vi "autoMaintainCurrentInstructions.vi"(6 "error in (no error)":errorcluster, 7 "MotionProfile acceleration":dbl[](array[numeric]), 8 "MotionProfile speed":dbl[](array[numeric]), 9 "running commands":string[][](array[string])) -> (0 "error out":errorcluster, 3 "running commands out":string[][](array[string]))   [LabVIEW 2013]
panel:
  out "BasicDriveOffset":dbl=1.07
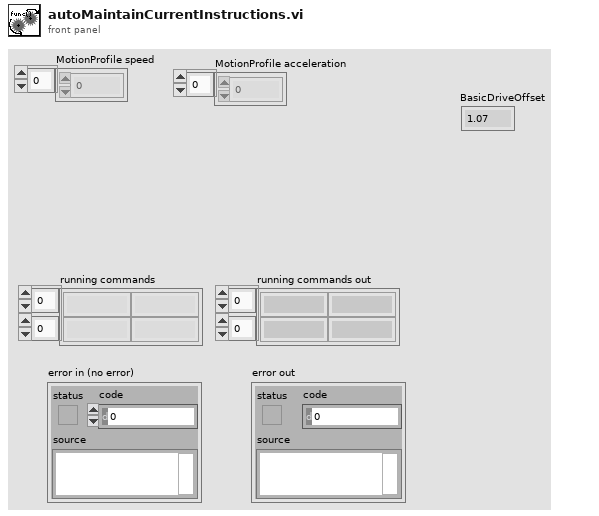
[diagram p1: front panel]
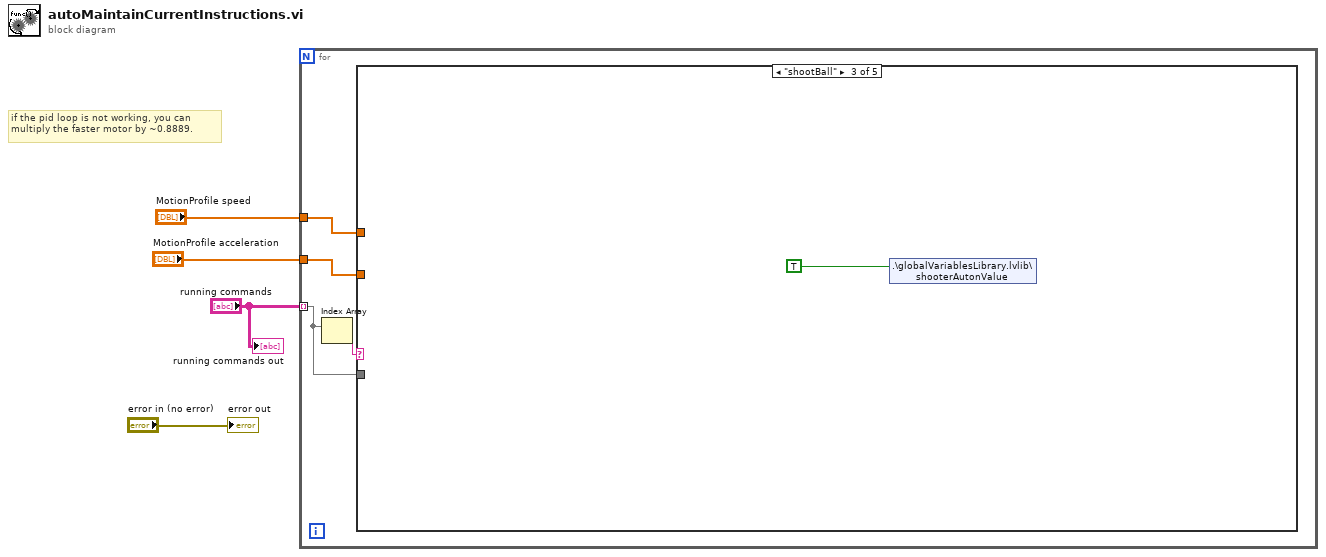
[diagram p0: block diagram]
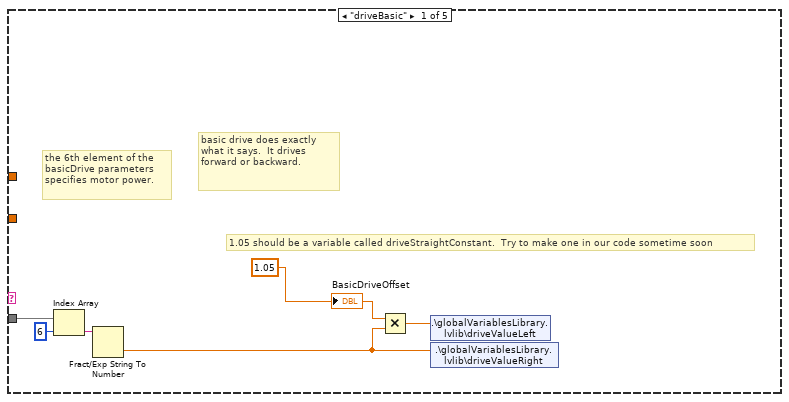
[diagram p2: hidden frame]
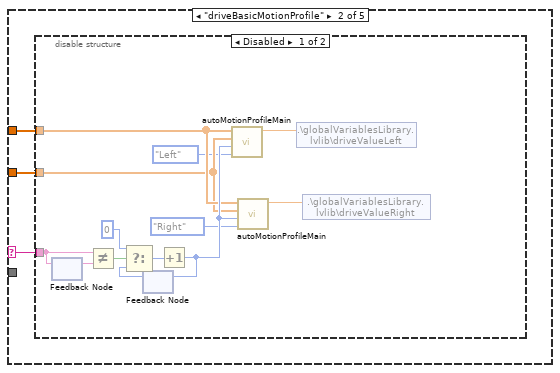
[diagram p3: hidden frame]
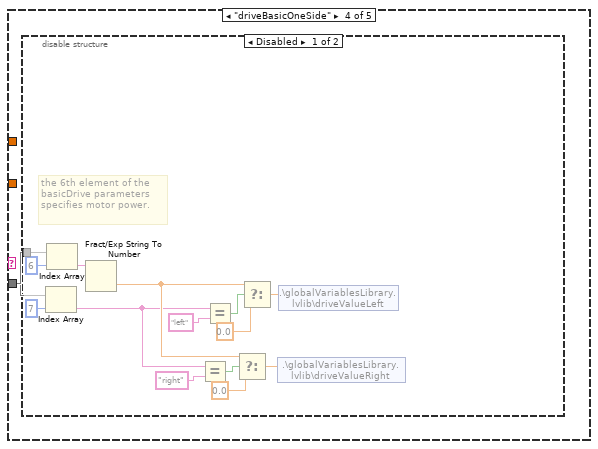
[diagram p5: hidden frame]
diagram:
  # "if the pid loop is not working, you can multiply the faster motor by ~0.8889."
  n1 = for {
    tunnel: "running commands" -> [w7] mode=indexing
    tunnel: "MotionProfile speed" -> [w6]
    tunnel: "MotionProfile acceleration" -> [w5]
    n2 = Index Array(array=w7) -> (element=w8:string)  [unwired: 1 in]
    n3 = case shown="\"shootBall\"" w8 {
      selector: w8 -> [_ w17 _ _ _]
      tunnel: w7 -> [w11 _ _ w32 _]
      tunnel: w6 -> [_ w16 _ _ _]
      tunnel: w5 -> [_ w15 _ _ _]
      frame "driveBasic" {
        w9 = 1.05
        # "1.05 should be a variable called driveStraightConstant.  Try to make one in our code sometime soon"
        # "basic drive does exactly what it says.  It drives forward or backward."
        # "the 6th element of the basicDrive parameters specifies motor power."
        n4 = Index Array(array=w11, index=6) -> (element=w13:string)
        n5 = Fract/Exp String To Number(string=w13) -> (number=w10:dbl)  [unwired: 3 in, 1 out]
        n6 = Multiply(x=w9, y=w10) -> (x*y=w12:dbl)
        n7 = shared-variable ".\\globalVariablesLibrary.lvlib\\driveValueLeft"(w12) -> ()  [unwired: 1 in, 1 out]
        n8 = shared-variable ".\\globalVariablesLibrary.lvlib\\driveValueRight"(w10) -> ()  [unwired: 1 in, 1 out]
        "BasicDriveOffset" <- w9
      }
      frame "driveBasicMotionProfile" {
        n9 = disable-structure shown="Disabled" {
          disable-tunnel: w17 -> [w30 _]
          disable-tunnel: w16 -> [w21 _]
          disable-tunnel: w15 -> [w20 _]
          frame Disabled {
            n10 = feedback #1() -> (w29:string)  [unwired: 1 in]
            n11 = feedback-in #1(w30) -> ()
            n12 = Not Equal?(x=w30, y=w29) -> (x != y?=w28:bool)
            n13 = feedback #2() -> (w25:i32)  [unwired: 1 in]
            n14 = Select(t=0, s=w28, f=w25) -> (s? t:f=w26:i32)
            n15 = Increment(x=w26) -> (x+1=w22:i32)
            n16 = feedback-in #2(w22) -> ()
            n17 = call "autoMotionProfileMain.vi"("Drivetrain Side"=enum16{"Left", "Right"}."Left", "Counter"=w22, "Acceleration steps"=w20, "Speed steps"=w21) -> ("MotorPower"=w24:dbl)  [unwired: 7 in]
            n18 = call "autoMotionProfileMain.vi"("Drivetrain Side"=enum16{"Left", "Right"}."Right", "Counter"=w22, "Acceleration steps"=w20, "Speed steps"=w21) -> ("MotorPower"=w23:dbl)  [unwired: 7 in]
            n19 = shared-variable ".\\globalVariablesLibrary.lvlib\\driveValueLeft"(w24) -> ()  [unwired: 1 in, 1 out]
            n20 = shared-variable ".\\globalVariablesLibrary.lvlib\\driveValueRight"(w23) -> ()  [unwired: 1 in, 1 out]
          }
          frame Enabled {
          }
        }
      }
      frame "shootBall" {
        n21 = shared-variable ".\\globalVariablesLibrary.lvlib\\shooterAutonValue"(TRUE) -> ()  [unwired: 1 in, 1 out]
      }
      frame "driveBasicOneSide" {
        n22 = disable-structure shown="Disabled" {
          disable-tunnel: w32 -> [w43 _]
          frame Disabled {
            # "the 6th element of the basicDrive parameters specifies motor power."
            n23 = Index Array(array=w43, index=7) -> (element=w34:string)
            n24 = Index Array(array=w43, index=6) -> (element=w46:string)
            n25 = Fract/Exp String To Number(string=w46) -> (number=w35:dbl)  [unwired: 3 in, 1 out]
            n26 = Equal?(x=w34, y="right") -> (x = y?=w33:bool)
            n27 = Equal?(x=w34, y="left") -> (x = y?=w41:bool)
            n28 = Select(t=w35, s=w33, f=0.0) -> (s? t:f=w36:dbl)
            n29 = Select(t=w35, s=w41, f=0.0) -> (s? t:f=w39:dbl)
            n30 = shared-variable ".\\globalVariablesLibrary.lvlib\\driveValueRight"(w36) -> ()  [unwired: 1 in, 1 out]
            n31 = shared-variable ".\\globalVariablesLibrary.lvlib\\driveValueLeft"(w39) -> ()  [unwired: 1 in, 1 out]
          }
          frame Enabled {
          }
        }
      }
      frame "testFunct", Default {
        # "This just acts as a time delay."
      }
    }
  }
  "running commands out" <- "running commands"
  "error out" <- "error in (no error)"
